vi "Requests.vi"(8 "error in (no error)":errorcluster, 9 "write enable":bool=TRUE, 11 "ICPCON ET-7051 in":refnum<class "ICPCON ET-7051.lvclass">) -> (0 "error out":errorcluster, 3 "ICPCON ET-7051 out":refnum<class "ICPCON ET-7051.lvclass">)   [LabVIEW 2021, in "ICPCON ET-7051.lvclass"]
uses:
  ICPCON ET-7051.lvclass
  D:/my_projects/projects/Algorithms/Labview/21/Modbus_v121c/Network Protocol/MB/Modbus Master CR.lvclass
  D:/my_projects/projects/Algorithms/Labview/21/Modbus_v121c/Network Protocol/Network Master/Network Master.lvclass
  MB/Modbus Master CR.lvclass/Modbus Master CR.ctl
  Modbus Data Unit/Modbus Data Unit.lvclass/Modbus Data Unit.ctl
  Network Master/Network Master.lvclass/Network Master.ctl
  Master Function Definition/Read Discrete Inputs Request.vi
  Network Master/Read write Master.vi
  Master Function Definition/Read Discrete Inputs Response.vi
  Modbus Data Unit/Construct PDU.vi
  Utility/Bytes to Bits.vi
  Master Function Definition/Function code mismatch error.vi
  Data Model/Error Generator.vi
  Modbus Data Unit/Deconstruct PDU.vi
  Modbus Data Unit/Modbus Data Unit.lvclass
  Data Model/Device Data Model.lvclass
  Transmission Data Unit/Transmission Data Unit.lvclass
  MB/Modbus Master CR.lvclass
  Network Master/Network Master.lvclass
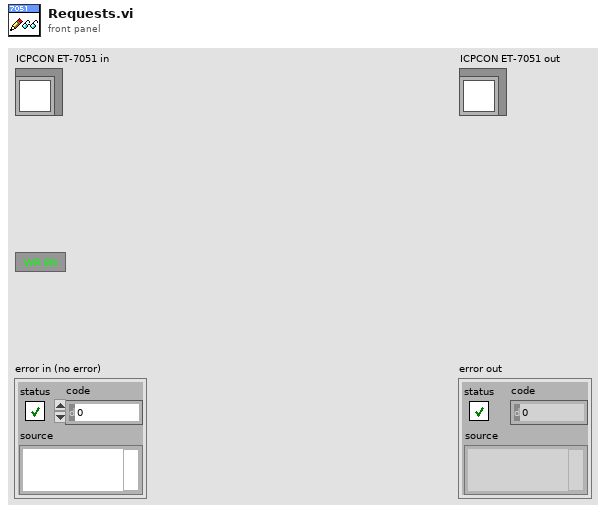
[diagram p1: front panel]
types:
  T1 = typedef "Modbus Master CR.lvclass/N channel.ctl" = cluster{"N DI channel":u16, "N DO channel":u16, "N AI channel":u16, "N AO channel":u16}
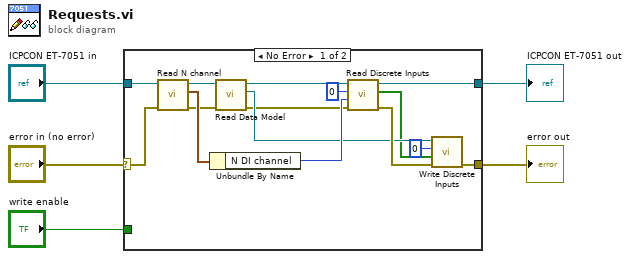
[diagram p0: block diagram]
diagram:
  n1 = case shown="No Error" "error in (no error)" {
    selector: "error in (no error)" -> [w17 w22]
    tunnel: [w13 w22] -> w3
    tunnel: [w6 w21] -> w4
    tunnel: "ICPCON ET-7051 in" -> [w19 w21]
    tunnel: "write enable" -> [_ _]
    frame No Error {
      n2 = call "Read N channel.vi"("error in (no error)"=w17, "MB_v2 in"=w19) -> ("error out"=w16:errorcluster, "N channel"=w20:T1, "MB_v2 out"=w18:refnum<class "ICPCON ET-7051.lvclass">)  [unwired: 7 in]
      n3 = Unbundle By Name(w20) -> ("N DI channel"=w14:u16)
      n4 = call "Read Data Model.vi"("error in (no error)"=w16, "MB_TCP in"=w18) -> ("error out"=w7:errorcluster, "Data Model"=w10:refnum<class "Device Data Model.lvclass">, "MB_TCP out"=w8:refnum<class "ICPCON ET-7051.lvclass">)  [unwired: 7 in]
      n5 = call "Read Discrete Inputs.vi"("error in (no error)"=w7, "number of discrete inputs"=w14, "starting address"=u16 0, "Modbus master in"=w8) -> ("error out"=w12:errorcluster, "discrete input values"=w9:bool[], "Modbus master out"=w6:refnum<class "ICPCON ET-7051.lvclass">)  [unwired: 5 in]
      n6 = call-dynamic "Write Discrete Inputs.vi"("error in (no error)"=w12, "input values"=w9, "starting address"=u16 0, "Device Data Model in"=w10) -> ("error out"=w13:errorcluster)  [unwired: 6 in, 1 out]
    }
    frame Error {
    }
  }
  "error out" <- w3
  "ICPCON ET-7051 out" <- w4
